vi "trplot_original.vi"(7 "Color_in":u32[](array[numeric]), 9 "scale":i32[](array[numeric]), 10 "T_in":dbl[][][](array[numeric]), 11 "XYGraph in":refnum<vi>) -> (3 "Plot_out":cluster{dbl[], dbl[]}[](array[cluster]))   [LabVIEW 2012]
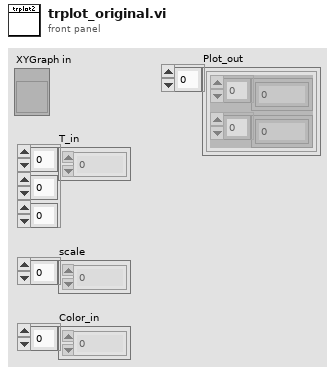
[diagram p1: front panel]
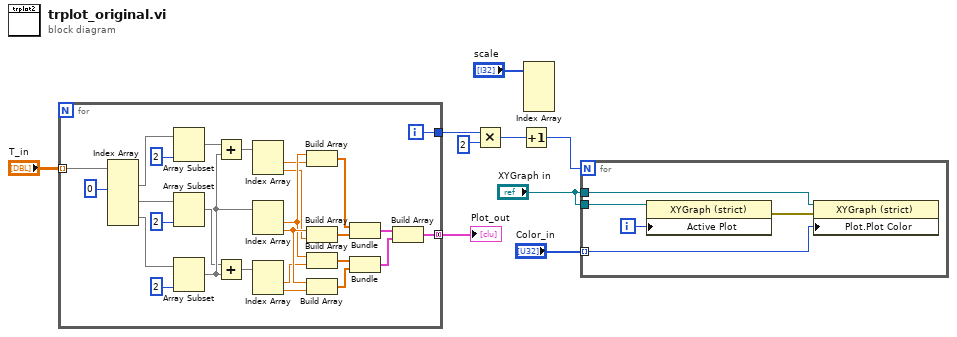
[diagram p0: block diagram]
diagram:
  n1 = for {
    tunnel: "T_in" -> [w16] mode=indexing
    tunnel: [w15] -> w3 mode=concatenating
    tunnel: [w14] -> w5
    i -> [w14]
    n2 = Index Array(array=w16, index (col) #1=0 ("disabled index (col)")) -> (element #1=w18:dbl[], element #2=w22:dbl[], element #3=w23:dbl[])  [unwired: 5 in]
    n3 = Array Subset(array=w18, length=2) -> (w26:dbl[])  [unwired: 1 in]
    n4 = Array Subset(array=w22, length=2) -> (w24:dbl[])  [unwired: 1 in]
    n5 = Array Subset(array=w23, length=2) -> (w25:dbl[])  [unwired: 1 in]
    n6 = Add(x=w26, y=w25) -> (x+y=w27:dbl[])
    n7 = Add(x=w24, y=w25) -> (x+y=w28:dbl[])
    n8 = Index Array(array=w27) -> (element #1=w13:dbl, element #2=w12:dbl)  [unwired: 2 in]
    n9 = Index Array(array=w25) -> (element #1=w35:dbl, element #2=w36:dbl)  [unwired: 2 in]
    n10 = Index Array(array=w28) -> (element #1=w11:dbl, element #2=w10:dbl)  [unwired: 2 in]
    n11 = Build Array(w35, w13) -> (w29:dbl[])
    n12 = Build Array(w36, w12) -> (w30:dbl[])
    n13 = Build Array(w35, w11) -> (w31:dbl[])
    n14 = Build Array(w36, w10) -> (w32:dbl[])
    n15 = Bundle(w29, w30) -> (w33:cluster{dbl[], dbl[]})  [unwired: 1 in]
    n16 = Bundle(w31, w32) -> (w34:cluster{dbl[], dbl[]})  [unwired: 1 in]
    n17 = Build Array(w33, w34) -> (w15:cluster{dbl[], dbl[]}[])
  }
  "Plot_out" <- w3
  n18 = Multiply(x=w5, y=2) -> (x*y=w7:i32)
  n19 = Increment(x=w7) -> (x+1=w8:i32)
  n20 = Index Array(array="scale") -> ()  [unwired: 4 in, 4 out]
  n21 = for {
    N: w8 -> [_]
    tunnel: "Color_in" -> [w39] mode=indexing
    tunnel: "XYGraph in" -> [w38]
    tunnel: "XYGraph in" -> [w37]
    i -> [w41]
    n22 = property on="Property Node" class="XYGraph (strict)"(reference=w38, "Active Plot"=w41) -> (error out=w40:errorcluster)  [unwired: 1 in, 1 out]
    n23 = property on="Property Node" class="XYGraph (strict)"(reference=w37, error in=w40, "Plot.Plot Color"=w39) -> ()  [unwired: 2 out]
  }
